vi "5_Difference_solution.vi"(10 "End (I8)":i8, 11 "Beginning (I8)":i8) -> (3 "Difference (I32)":i32)   [LabVIEW 2014]
panel:
  # "Example:"
  # "Beginning"
  # "End"
  # "Difference"
  # "0"
  # "2"
  # "4"
  # "-5"
  # "-4"
  # "40"
  # "10"
  # "13"
  # "1582"
  # "4"
  # "100"
  # "25103600"
  # "Calculate the difference \nrefer to the example"
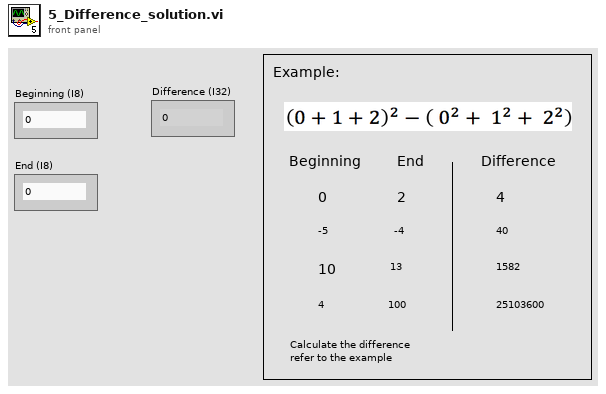
[diagram p1: front panel]
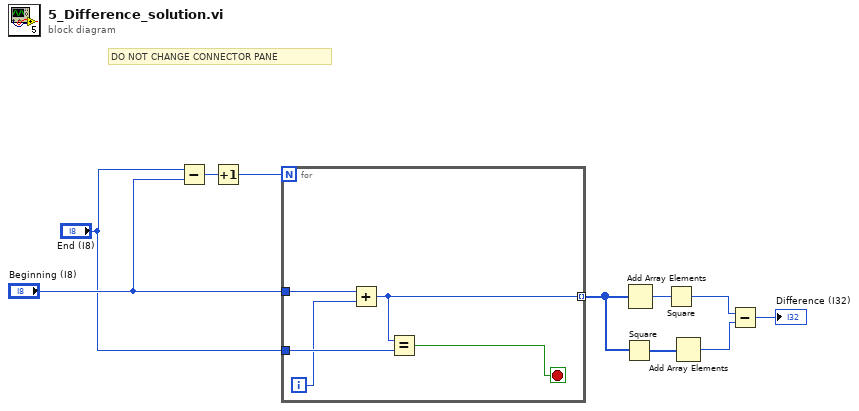
[diagram p0: block diagram]
diagram:
  # "DO NOT CHANGE CONNECTOR PANE"
  n1 = Subtract(x="End (I8)", y="Beginning (I8)") -> (x-y=w10:i8)
  n2 = Increment(x=w10) -> (x+1=w9:i8)
  n3 = for {
    N: w9 -> [_]
    tunnel: "Beginning (I8)" -> [w15]
    tunnel: "End (I8)" -> [w13]
    tunnel: [w11] -> w5 mode=indexing
    i -> [w12]
    stop <- w14 stop-if-true
    n4 = Add(x=w15, y=w12) -> (x+y=w11:i32)
    n5 = Equal?(x=w11, y=w13) -> (x = y?=w14:bool)
  }
  n6 = Square(x=w5) -> (x^2=w4:i32[])
  n7 = Add Array Elements(numeric array=w5) -> (sum=w6:i32)
  n8 = Square(x=w6) -> (x^2=w3:i32)
  n9 = Add Array Elements(numeric array=w4) -> (sum=w2:i32)
  n10 = Subtract(x=w3, y=w2) -> (x-y=→"Difference (I32)":i32)
